vi "Temperature Limit.vi"() -> ()   [LabVIEW 2022 SP3]
doc: "This VI simulates the acquisition of temperature, graphs the temperature, and notifies the user if the temperature is over the limit."
panel:
  in  "Start":bool
  in  "Delta t (ms)":i32(slide)=400 scale=50.0..500.0
  in  "Stop":bool
  in  "High Limit":dbl=28.0 format="%.2f"
  out "Temperature":cluster{"Temperature":dbl, "High Limit":dbl}(graph)={"Temperature"=85.88749999999999, "High Limit"=80.0}
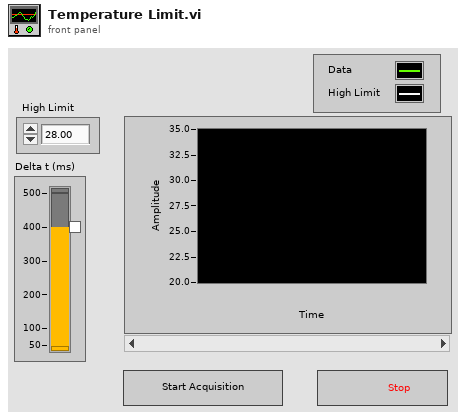
[diagram p1: front panel]
types:
  T1 = enum8{"Enabled", "Disabled", "Disabled and Grayed Out"}
  T2 = cluster{"Temperature Value":dbl, "High Limit":dbl}
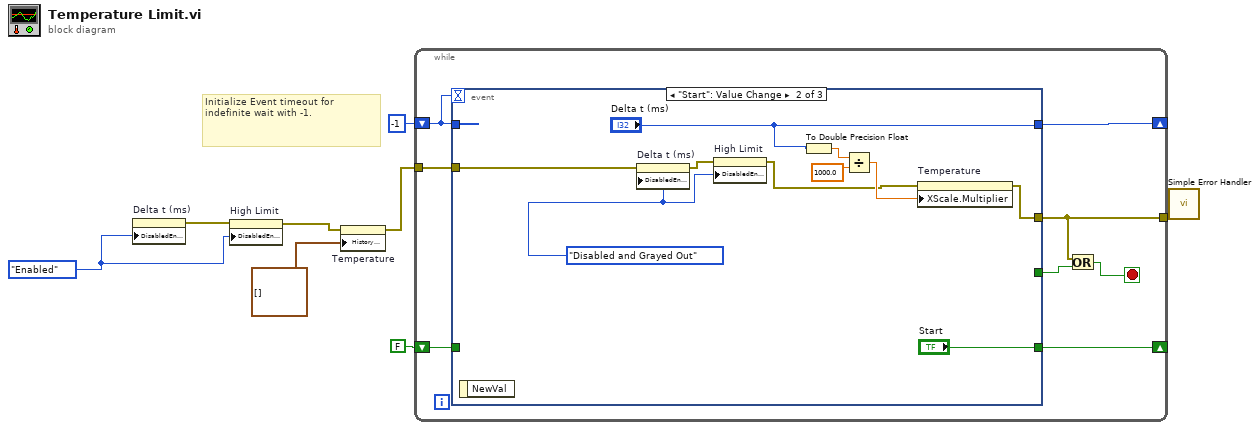
[diagram p0: block diagram]
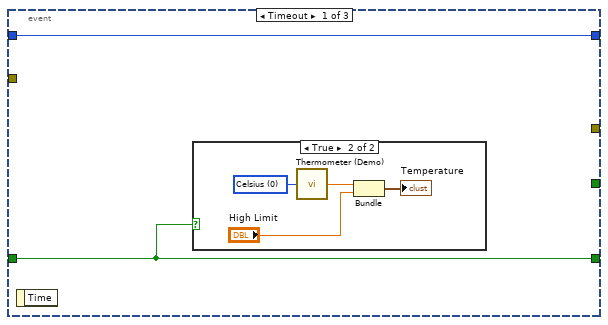
[diagram p2: hidden frame]
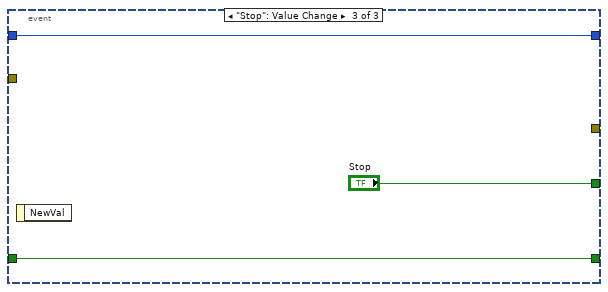
[diagram p4: hidden frame]
diagram:
  w5 = T1."Enabled" ("Disabled")
  # "Initialize Event timeout for indefinite wait with -1."
  n1 = property on="Delta t (ms)" class="Slide (strict)"("DisabledEnum"=w5) -> (error out=w4:errorcluster)  [unwired: 2 in, 1 out]
  n2 = property on="High Limit" class="DigNum (strict)"(error in=w4, "DisabledEnum"=w5) -> (error out=w2:errorcluster)  [unwired: 1 in, 1 out]
  n3 = property on="Temperature" class="WFChart (strict)"(error in=w2, "History Data"=cluster{"Temperature":dbl, "High Limit":dbl}[] []) -> (error out=w1:errorcluster)  [unwired: 1 in, 1 out]
  n4 = while {
    tunnel: [w11] -> w7
    shift-right: [w15] -> _
    shift-left: FALSE ("Start") -> [w14]
    shift-right: [w13] -> _
    shift-left: -1 ("Delta t (ms)") -> [w9]
    tunnel: w1 -> [w12]
    stop <- w10 stop-if-true
    n5 = event shown="[1] \"Start\": Value Change" {
      selector: _ -> [_ _ _]
      dyn-events: _ -> [_ _ _]
      timeout: w9 -> [_ _ _]
      tunnel: [_ _ "Stop"] -> w16
      tunnel: [_ w23 _] -> w11
      tunnel: [w17 "Start" w34] -> w15
      tunnel: w14 -> [w17 _ w34]
      tunnel: [w18 "Delta t (ms)" w33] -> w13
      tunnel: w9 -> [w18 _ w33]
      tunnel: w12 -> [_ w30 _]
      event Timeout {
        n6 = event-data() -> ()  [unwired: 1 in, 1 out]
        n7 = case shown="True" w17 {
          frame False {
          }
          frame True {
            w19 = u16 0 items=["Celsius", "Fahrenheit"] ("Units (0: Celsius)")
            n8 = call "Thermometer (Demo).vi"("Units (0: Celsius)"=w19) -> ("Temperature Value"=w20:dbl)
            n9 = Bundle("Temperature Value"=w20, "High Limit"="High Limit") -> (→"Temperature":T2)  [unwired: 1 in]
          }
        }
      }
      event "Start": Value Change {
        w31 = T1."Disabled and Grayed Out" ("Disabled")
        n10 = event-data() -> ()  [unwired: 1 in, 1 out]
        n11 = property on="Delta t (ms)" class="Slide (strict)"(error in=w30, "DisabledEnum"=w31) -> (error out=w25:errorcluster)  [unwired: 1 in, 1 out]
        n12 = property on="High Limit" class="DigNum (strict)"(error in=w25, "DisabledEnum"=w31) -> (error out=w24:errorcluster)  [unwired: 1 in, 1 out]
        n13 = To Double Precision Float(number="Delta t (ms)") -> (double precision float=w28:dbl)
        n14 = Divide(x=w28, y=1000.0) -> (x/y=w26:dbl)
        n15 = property on="Temperature" class="WFChart (strict)"(error in=w24, "XScale.Multiplier"=w26) -> (error out=w23:errorcluster)  [unwired: 1 in, 1 out]
      }
      event "Stop": Value Change {
        n16 = event-data() -> ()  [unwired: 1 in, 1 out]
      }
    }
    n17 = Or(x=w11, y=w16) -> (x .or. y?=w10:bool)
  }
  n18 = call <vilib>:"Simple Error Handler.vi"("error in (no error)"=w7) -> ()  [unwired: 4 in, 5 out]
